vi "AVS_GetParameter.vi"(0 "a_hDevice":i32, 7 "a_Size":u32, 9 "RequiredSizeInput":u32, 11 "DeviceParm":u8[](array[numeric])) -> (4 "Output Value":i32, 10 "RequiredSizeOutput":u32, 15 "DeviceParam":u8[](array[numeric]))   [LabVIEW 2016]
uses:
  libavs.so
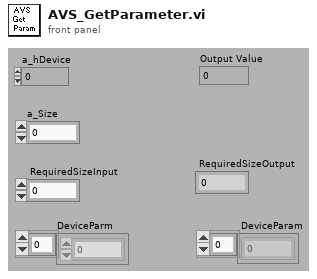
[diagram p1: front panel]
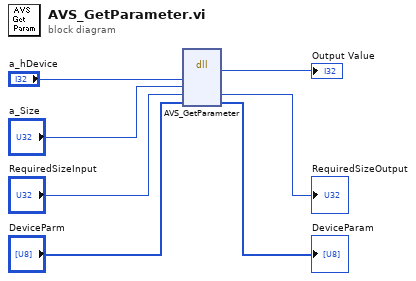
[diagram p0: block diagram]
diagram:
  n1 = dll-call lib="home/harini/tcs/ts_sedspectrometer/ss_sedspectrometer/VIs/libavs.so" fn="AVS_GetParameter"("a_hDevice"="a_hDevice", "a_Size"="a_Size", "a_pRequiredSize"="RequiredSizeInput", "a_pDeviceParm"="DeviceParm") -> ("return type"=→"Output Value":i32, "a_pRequiredSize"=→"RequiredSizeOutput":u32, "a_pDeviceParm"=→"DeviceParam":u8[])  [unwired: 5 in, 2 out]
